vi "Lian_Lab03_I.vi"() -> ()   [LabVIEW 2020]
panel:
  out "Waveform Graph":dbl[](graph)
  out "Iteration Count":i32
  out "Waveform Chart":dbl[](graph)
  in  "Scale Factor":dbl
  in  "Phase":dbl
  in  "Offset":dbl
  in  "Amplitude":dbl=2.0
  in  "Frequency":dbl=20.0
  in  "Scale Data?":bool
  out "Iteration Count":i32
  in  "Scale Factor":dbl
  in  "Phase":dbl
  in  "Amplitude":dbl=2.0
  in  "Frequency":dbl=20.0
  in  "Offset":dbl
  in  "Scale Data?":bool
  out "Waveform Graph":dbl[](graph)
  out "Waveform Chart":dbl[](graph)
  # "Method 2"
  # "Note: Data generated from \"concatenating tunnel\""
  # "Method 1"
  # "Note: Data generated from shift register"
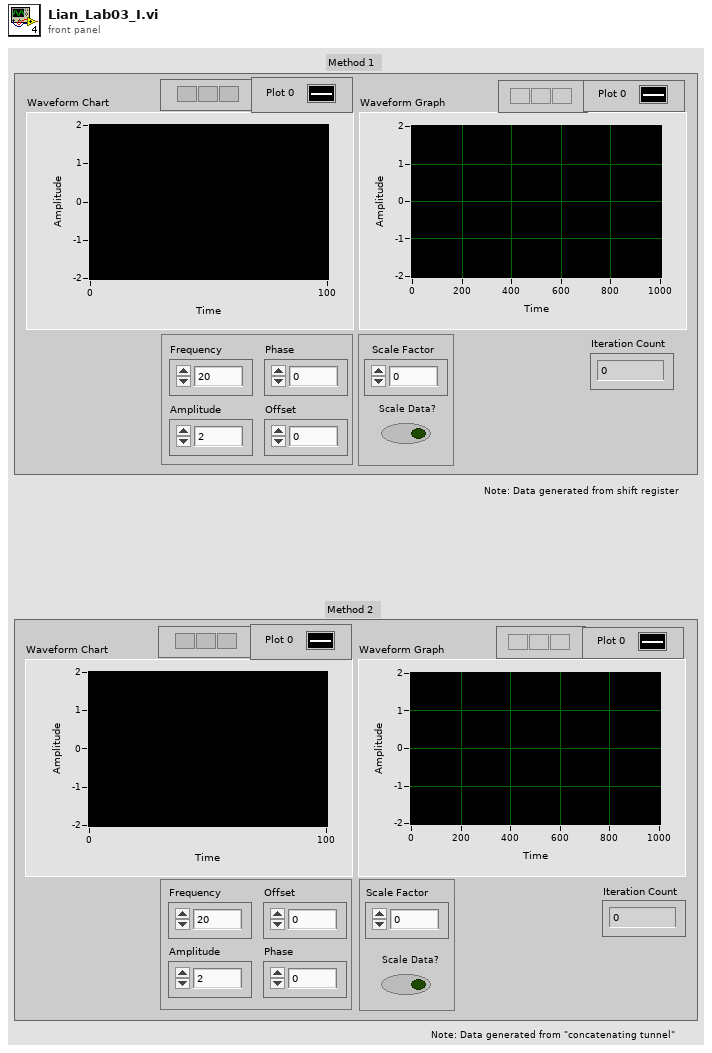
[diagram p1: front panel]
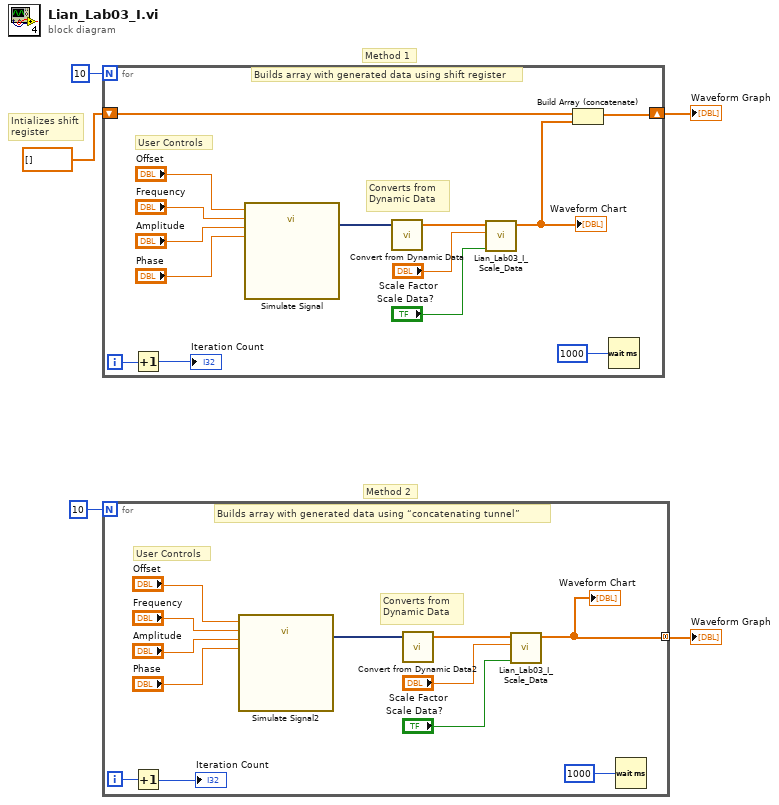
[diagram p0: block diagram]
diagram:
  # "Intializes shift\nregister"
  # "Method 2"
  # "Method 1"
  n1 = for {
    N: 10 -> [_]
    shift-right: [w16] -> w2
    shift-left: dbl[] [] -> [w17]
    i -> [w14]
    # "User Controls"
    # "Builds array with generated data using shift register"
    # "Converts from \nDynamic Data"
    n2 = Increment(x=w14) -> (x+1=→"Iteration Count":i32)
    n3 = call "Simulate Signal"("Offset"="Offset", "Frequency"="Frequency", "Amplitude"="Amplitude", "Phase"="Phase") -> ("Sine"=w18:dynamicdata)  [unwired: 10 in, 1 out]
    n4 = call "Convert from Dynamic Data"("Dynamic Data Type"=w18) -> ("Array"=w15:dbl[])  [unwired: 3 in]
    n5 = call "Lian_Lab03_I_Scale_Data.vi"("Boolean"="Scale Data?", "Scale Factor"="Scale Factor", "Input Array"=w15) -> ("Output Array"=w6:dbl[])  [unwired: 8 in]
    "Waveform Chart" <- w6
    n6 = Build Array (concatenate) "Build Array"(w17, w6) -> (w16:dbl[])
    n7 = Wait (ms)(milliseconds to wait=u32 1000) -> ()  [unwired: 1 out]
  }
  "Waveform Graph" <- w2
  n8 = for {
    N: 10 -> [_]
    tunnel: [w20] -> w1 mode=concatenating
    i -> [w28]
    # "User Controls"
    # "Builds array with generated data using “concatenating tunnel”"
    # "Converts from \nDynamic Data"
    n9 = Increment(x=w28) -> (x+1=→"Iteration Count":i32)
    n10 = call "Simulate Signal2"("Offset"="Offset", "Frequency"="Frequency", "Amplitude"="Amplitude", "Phase"="Phase") -> ("Sine"=w30:dynamicdata)  [unwired: 10 in, 1 out]
    n11 = call "Convert from Dynamic Data2"("Dynamic Data Type"=w30) -> ("Array"=w29:dbl[])  [unwired: 3 in]
    n12 = call "Lian_Lab03_I_Scale_Data.vi"("Boolean"="Scale Data?", "Scale Factor"="Scale Factor", "Input Array"=w29) -> ("Output Array"=w20:dbl[])  [unwired: 8 in]
    "Waveform Chart" <- w20
    n13 = Wait (ms)(milliseconds to wait=u32 1000) -> ()  [unwired: 1 out]
  }
  "Waveform Graph" <- w1
